vi "sandbox.vi"() -> ()   [LabVIEW 2020]
uses:
  orderbook/orderbook.command.ctl
  orderbook/orderbook.command.type.ctl
panel:
  out "length":i32
  out "*(type *) &x":string
  out "data string":string
  out "type string":i16[](array[numeric])
  out "data":T1
  out "variant":variant
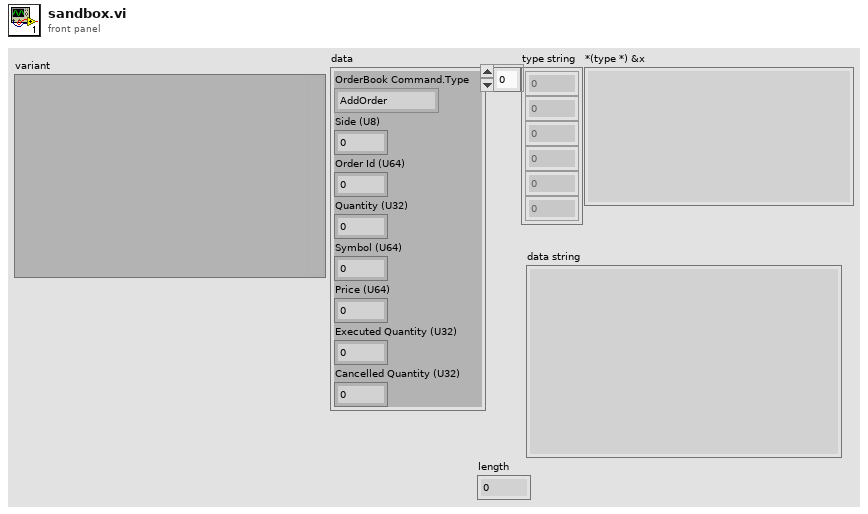
[diagram p1: front panel]
types:
  T1 = typedef "orderbook.command.ctl" = cluster{"OrderBook Command.Type":T2, "Side (U8)":u8, "Order Id (U64)":u64, "Quantity (U32)":u32, "Symbol (U64)":u64, "Price (U64)":u64, "Executed Quantity (U32)":u32, "Cancelled Quantity (U32)":u32}
  T2 = typedef "orderbook.command.type.ctl" = enum16{"AddOrder", "OrderExecuted", "ReduceSize", "ModifyOrder", "DeleteOrder", "Query"}
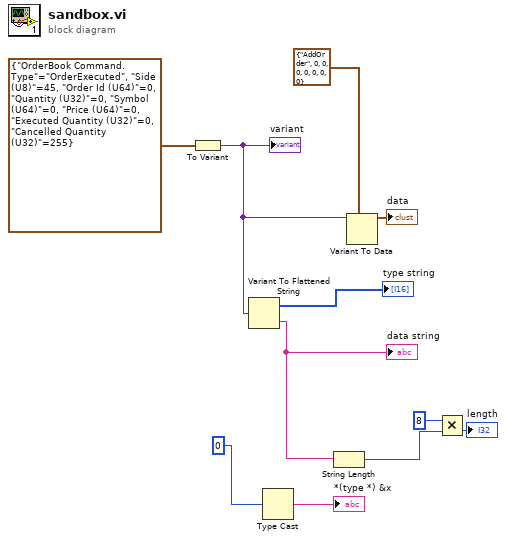
[diagram p0: block diagram]
diagram:
  n1 = To Variant(anything=T1 {"OrderBook Command.Type"=enum."OrderExecuted", "Side (U8)"=45, "Order Id (U64)"=0, "Quantity (U32)"=0, "Symbol (U64)"=0, "Price (U64)"=0, "Executed Quantity (U32)"=0, "Cancelled Quantity (U32)"=255} ("Cluster")) -> (Variant=w9:variant)
  "variant" <- w9
  n2 = Variant To Flattened String(Variant=w9) -> (data string=w3:string, 1:→"type string":i16[])
  "data string" <- w3
  n3 = Type Cast(x=u8 0) -> (*(type *) &x=→"*(type *) &x":string)  [unwired: 1 in]
  n4 = String Length(string=w3) -> (length=w5:i32)
  n5 = Variant To Data(type=T1 {"OrderBook Command.Type"=enum."AddOrder", "Side (U8)"=0, "Order Id (U64)"=0, "Quantity (U32)"=0, "Symbol (U64)"=0, "Price (U64)"=0, "Executed Quantity (U32)"=0, "Cancelled Quantity (U32)"=0} ("Cluster"), Variant=w9) -> (data=→"data":T1)  [unwired: 1 in, 1 out]
  n6 = Multiply(x=8, y=w5) -> (x*y=→"length":i32)
